vi "Keithley J-t List_IIT.vi"(0 "VISA resource name in":refnum<visa-resource-name>, 9 "Voltage List":dbl[](array[numeric]), 11 "error in (no error)":errorcluster) -> (4 "VISA resource name out":refnum<visa-resource-name>, 6 "Data Array":dbl[][](array[numeric]), 15 "Measurement Complete":bool)   [LabVIEW 2011]
doc: "Configures a sweep and takes voltage and current readings at each point."
uses:
  <instrlib>/Keithley 24XX/Public/Data/Read (Multiple Points).vi
  <instrlib>/Keithley 24XX/Keithley 24XX.lvlib
panel:
  in  "Source Mode  (0: Voltage)":u16(ring) items=["Voltage", "Current"]
  # "(c) 2006 National Instruments.  ALL RIGHTS RESERVED."
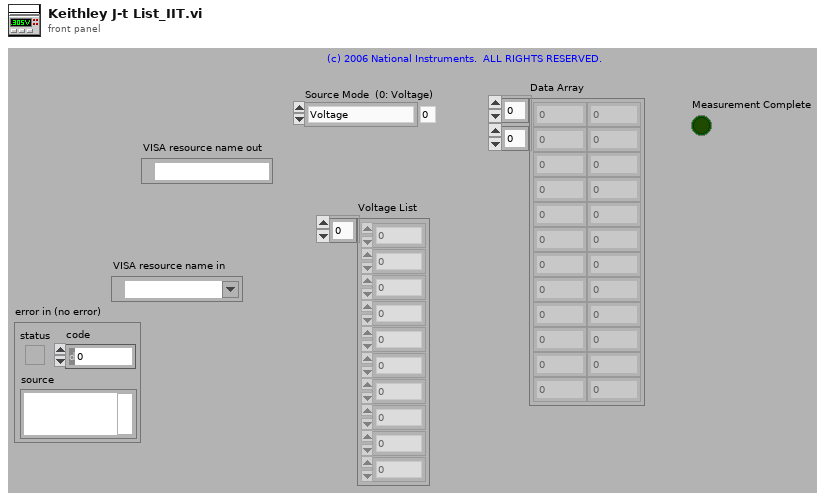
[diagram p1: front panel]
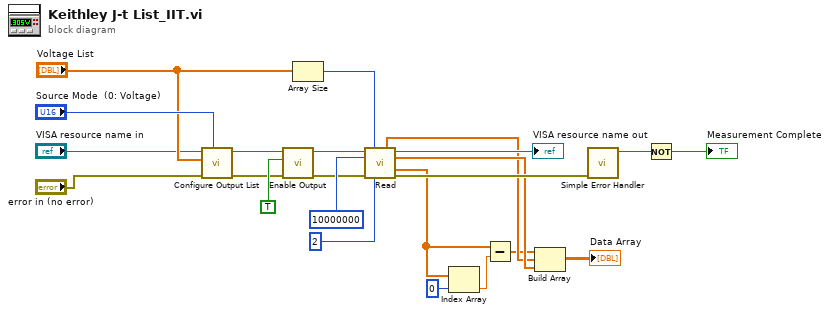
[diagram p0: block diagram]
diagram:
  n1 = call <instrlib>:"Configure Output List.vi"("Source Mode  (0: Voltage)"="Source Mode  (0: Voltage)", "error in (no error)"="error in (no error)", "Output List"="Voltage List", "VISA resource name"="VISA resource name in") -> ("error out"=w5:errorcluster, "VISA resource name out"=w6:refnum<visa-resource-name>)  [unwired: 6 in]
  n2 = call <instrlib>:"Enable Output.vi"("error in (no error)"=w5, "Enable Output (T: Enable)"=TRUE ("Output (Off)"), "VISA resource name"=w6) -> ("error out"=w3:errorcluster, "VISA resource name out"=w4:refnum<visa-resource-name>)  [unwired: 7 in]
  n3 = Array Size(array="Voltage List") -> (size(s)=w13:i32)
  n4 = call-poly <instrlib>:"Read.vi"("VISA resource name"=w4, "Sample Count (1)"=w13, "Timeout (10000 ms)"=10000000, "error in (no error)"=w3, "Output Mode (0: Fixed)"=2) -> ("Voltage"=w12:sgl[], "VISA resource name out"=→"VISA resource name out":refnum<visa-resource-name>, "Current"=w15:sgl[], "Timestamp"=w9:sgl[], "error out"=w23:errorcluster)  [unwired: 4 in, 2 out]
  n5 = Index Array(array=w9, index=0) -> (element=w11:sgl)
  n6 = Subtract(x=w9, y=w11) -> (x-y=w10:sgl[])
  n7 = Build Array(w10, w12, w15) -> (→"Data Array":sgl[][])
  n8 = call <vilib>:"Simple Error Handler.vi"("error in (no error)"=w23) -> ("error?"=w21:bool)  [unwired: 4 in, 4 out]
  n9 = Not(x=w21) -> (.not. x?=→"Measurement Complete":bool)
